vi "lockin_config(SubVI).vi"(0 "VISA Refnum in":refnum<visa-resource-name>, 1 "Enable Sync Filter (F: Disable)":bool, 2 "Input Shield Grounding (0: Float)":u16, 3 "Low Pass Filter Slope (1: 12dB/oct)":u16, 4 "Internal Reference Frequency (1000 Hz)":dbl, 5 "error in (no error)":errorcluster, 6 "Input Notch Filter (0: None)":u16, 7 "Dynamic Reserve (-1: Auto Reserve)":i16, 8 "Input Coupling (0: AC)":u16, 9 "Sensitivity (-1: Auto gain)":i16, 10 "Input Connection (0: Single-Ended Voltage)":u16, 11 "Time Constant (8: 100ms)":u16) -> (14 "VISA Refnum out":refnum<visa-resource-name>, 19 "error out":errorcluster)   [LabVIEW 2019]
uses:
  National Instruments/LabVIEW 2019/instr.lib/Stanford Research 830/Stanford Research 830.lvlib
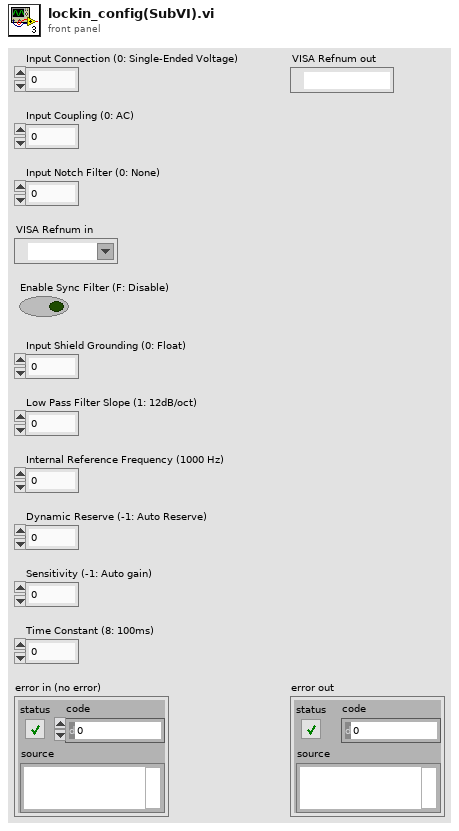
[diagram p1: front panel]
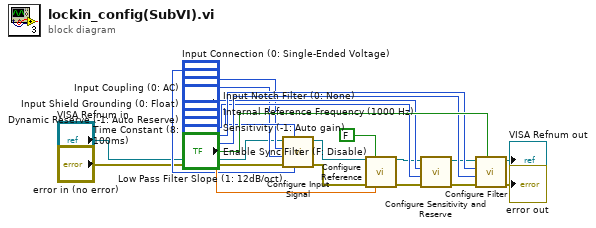
[diagram p0: block diagram]
diagram:
  n1 = call "Configure Input Signal.vi"("Input Notch Filter (0: None)"="Input Notch Filter (0: None)", "Input Shield Grounding (0: Float)"="Input Shield Grounding (0: Float)", "error in (no error)"="error in (no error)", "Input Coupling (0: AC)"="Input Coupling (0: AC)", "Input Connection (0: Single-Ended Voltage)"="Input Connection (0: Single-Ended Voltage)", "VISA resource name"="VISA Refnum in") -> ("error out"=w4:errorcluster, "VISA resource name out"=w3:refnum<visa-resource-name>)  [unwired: 4 in]
  n2 = call "Configure Reference.vi"("VISA resource name"=w3, "Auto Phase (T: Enabled)"=FALSE, "error in (no error)"=w4, "Internal Reference Frequency (1000 Hz)"="Internal Reference Frequency (1000 Hz)") -> ("VISA resource name out"=w6:refnum<visa-resource-name>, "error out"=w7:errorcluster)  [unwired: 10 in]
  n3 = call "Configure Sensitivity and Reserve.vi"("error in (no error)"=w7, "Sensitivity (-1: Auto gain)"="Sensitivity (-1: Auto gain)", "Dynamic Reserve (-1: Auto Reserve)"="Dynamic Reserve (-1: Auto Reserve)", "VISA resource name"=w6) -> ("error out"=w9:errorcluster, "VISA resource name out"=w8:refnum<visa-resource-name>)  [unwired: 6 in]
  n4 = call "Configure Filter.vi"("Enable Sync Filter (F: Disable)"="Enable Sync Filter (F: Disable)", "error in (no error)"=w9, "Low Pass Filter Slope (1: 12dB/oct)"="Low Pass Filter Slope (1: 12dB/oct)", "Time Constant (8: 100ms)"="Time Constant (8: 100ms)", "VISA resource name"=w8) -> ("error out"=→"error out":errorcluster, "VISA resource name out"=→"VISA Refnum out":refnum<visa-resource-name>)  [unwired: 5 in]
